vi "sync init.vi"(8 "error in (no error)":errorcluster, 9 "data allocations in":T1, 10 "shared memory configuration in":refnum<class "Shared Memory configuration.lvclass">, 11 "shared memory runtime in":refnum<class "Shared Memory runtime.lvclass">) -> (0 "error out":errorcluster, 1 "data allocations out":T1, 2 "shared memory configuration out":refnum<class "Shared Memory configuration.lvclass">, 3 "shared memory runtime out":refnum<class "Shared Memory runtime.lvclass">)   [LabVIEW 2014, in "Shared Memory runtime.lvclass"]
uses:
  Shared Memory runtime.lvclass
  configuration/Shared Memory configuration.lvclass
  <vilib>/NI/Tag Bus Module Framework/channel/data tables.ctl
  <vilib>/NI/Tag Bus/dictionary/data dictionary.lvclass
  <vilib>/NI/Tag Bus/dictionary table pair.ctl
  <vilib>/NI/Tag Bus/table/data table.ctl
  configuration/Shared Memory configuration.lvclass/Shared Memory configuration.ctl
  controls/sync data.ctl
  controls/semaphore data.ctl
  <vilib>/NI/NI Linux RT IPC/POSIX Threads/Classes/Semaphore/Controls/reference.ctl
  <vilib>/NI/NI Linux RT IPC/POSIX Threads/Classes/Semaphore/Semaphore.lvclass
  <vilib>/NI/NI Linux RT IPC/Shared Memory/Classes/Shared Memory/Public/Controls/reference.ctl
  <vilib>/NI/NI Linux RT IPC/Shared Memory/Classes/Shared Memory/Shared Memory.lvclass
  controls/sync timing indices.ctl
  controls/sync timing pointers.ctl
  Shared Memory runtime.lvclass/Shared Memory runtime.ctl
  configuration/Read sync enable.vi
  configuration/Read sync shm name.vi
  configuration/Read include start time.vi
  configuration/Read sync start of cycle.vi
  configuration/Read sync end of cycle.vi
  configuration/Read sync timeout seconds.vi
  Write sync data.vi
  <vilib>/NI/Tag Bus/table/data table.lvlib
  <vilib>/NI/Tag Bus/tag bus.lvlib
  <vilib>/NI/Tag Bus Module Framework/channel/TBM channel.lvclass
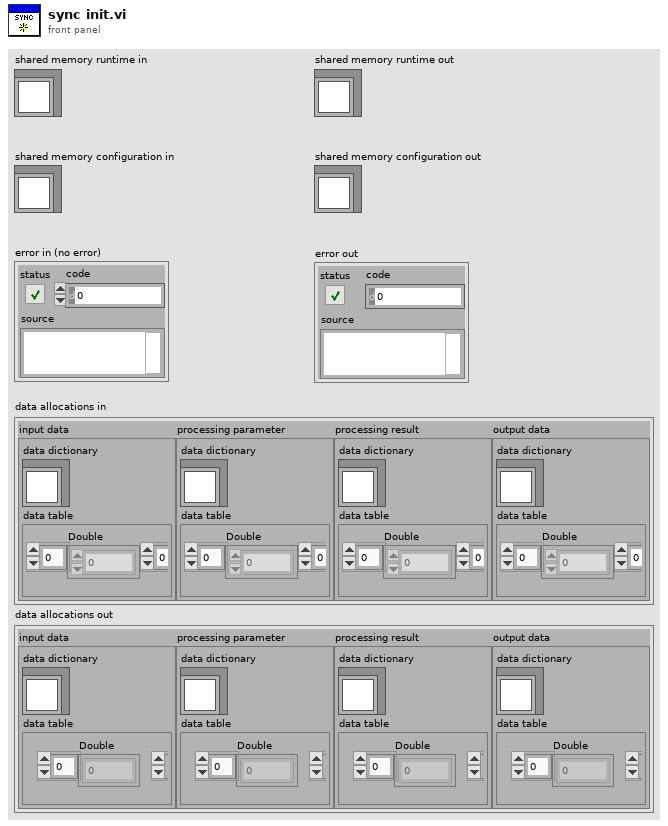
[diagram p1: front panel]
types:
  T1 = typedef "TBM channel.lvclass/data tables.ctl" = cluster{"input data":T2, "processing parameter":T2, "processing result":T2, "output data":T2}
  T2 = typedef "tag bus.lvlib/dictionary table pair.ctl" = cluster{"data dictionary":refnum<class "data dictionary.lvclass">, "data table":T3}
  T3 = typedef "tag bus.lvlib/data table.lvlib/data table.ctl" = cluster{"Double":dbl[], "Single":sgl[], "I64":i64[], "I32":i32[], "I16":i16[], "I8":i8[], "U64":u64[], "U32":u32[], "U16":u16[], "U8":u8[], "Boolean":bool[], "String":string[], "Array of Double":cluster{"DBL Array":dbl[]}[], "Array of Single":cluster{"SGL Array":sgl[]}[], "Array of I64":cluster{"I64 Array":i64[]}[], "Array of I32":cluster{"I32 Array":i32[]}[], "Array of I16":cluster{"I16 Array":i16[]}[], "Array of I8":cluster{"I8 Array":i8[]}[], "Array of U64":cluster{"U64 Array":u64[]}[], "Array of U32":cluster{"U32 Array":u32[]}[], "Array of U16":cluster{"U16 Array":u16[]}[], "Array of U8":cluster{"U8 Array":u8[]}[], "Array of Boolean":cluster{"Boolean Array":bool[]}[], "Array of String":cluster{"String Array":string[]}[]}
  T4 = typedef "Shared Memory configuration.lvclass/sync item.ctl" = cluster{"mechanism":T5, "name":string}
  T5 = typedef "Shared Memory configuration.lvclass/sync mechanism.ctl" = enum16{"Semaphore"}
  T6 = typedef "Shared Memory runtime.lvclass/sync data.ctl" = cluster{"semaphores soc":T7[], "semaphores eoc":T7[], "timeout":dbl, "enabled":bool, "sync shared memory":T9, "publish timing":bool, "timing indices":T10, "timing pointers":T11}
  T7 = typedef "Shared Memory runtime.lvclass/semaphore data.ctl" = cluster{"semaphore":T8, "name":string}
  T8 = typedef "POSIX Threads.lvlib/Semaphore.lvclass/reference.ctl" = refnum<data-value>
  T9 = typedef "Shared Memory.lvlib/Shared Memory.lvclass/reference.ctl" = refnum<data-value>
  T10 = typedef "Shared Memory runtime.lvclass/sync timing indices.ctl" = cluster{"start time index":i32}
  T11 = typedef "Shared Memory runtime.lvclass/sync timing pointers.ctl" = cluster{"start sec ptr":u64, "start nsec ptr":u64}
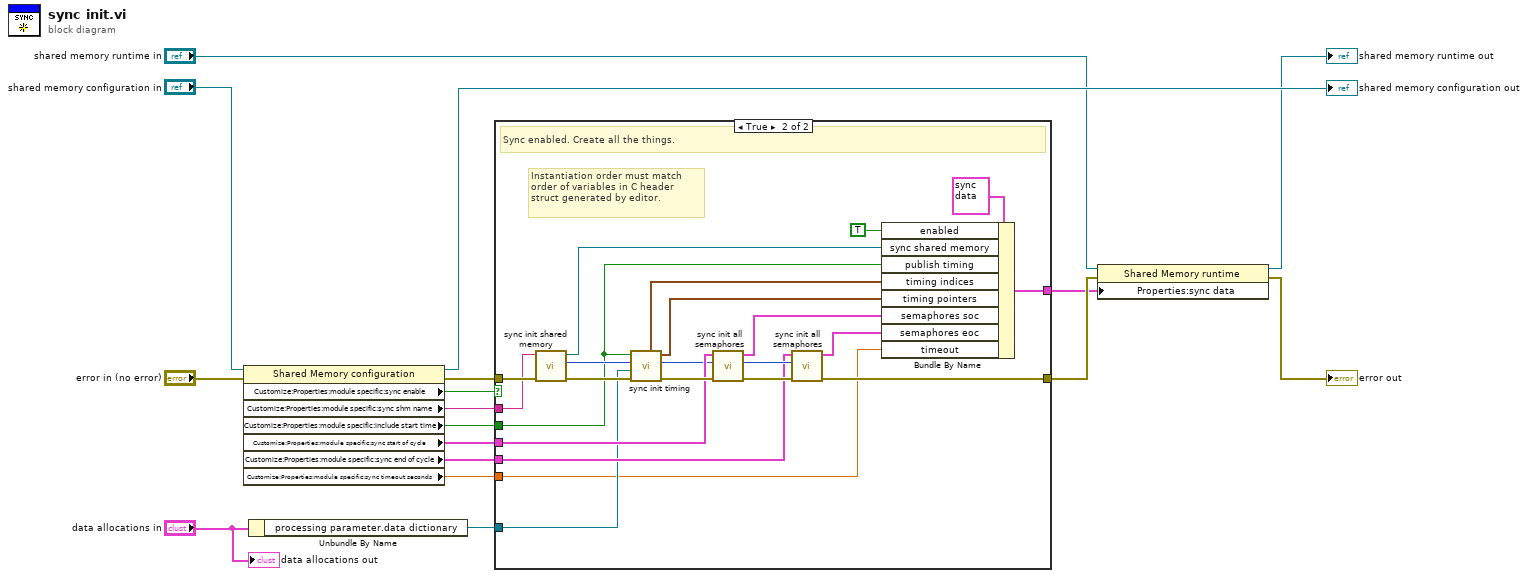
[diagram p0: block diagram]
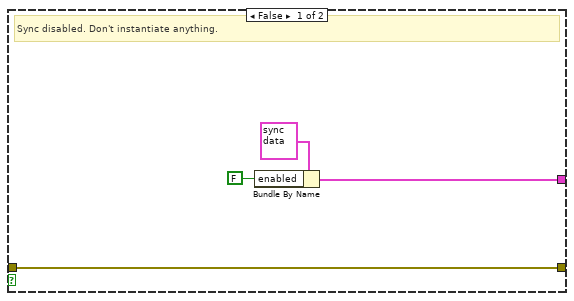
[diagram p2: hidden frame]
diagram:
  n1 = property class="Shared Memory configuration"(reference="shared memory configuration in", error in="error in (no error)") -> (reference out=→"shared memory configuration out":refnum<class "Shared Memory configuration.lvclass">, error out=w12:errorcluster, "Customize:Properties:module specific:sync enable"=w7:bool, "Customize:Properties:module specific:sync shm name"=w10:string, "Customize:Properties:module specific:include start time"=w3:bool, "Customize:Properties:module specific:sync start of cycle"=w9:T4[], "Customize:Properties:module specific:sync end of cycle"=w8:T4[], "Customize:Properties:module specific:sync timeout seconds"=w4:dbl)
  n2 = Unbundle By Name("data allocations in") -> ("processing parameter.data dictionary"=w1:refnum<class "data dictionary.lvclass">)
  n3 = case shown="True" w7 {
    tunnel: w12 -> [w21 w43]
    tunnel: [w21 w32] -> w17
    tunnel: w10 -> [_ w42]
    tunnel: w9 -> [_ w29]
    tunnel: w8 -> [_ w34]
    tunnel: [w18 w40] -> w6
    tunnel: w4 -> [_ w22]
    tunnel: w3 -> [_ w26]
    tunnel: w1 -> [_ w27]
    frame False {
      # "Sync disabled. Don't instantiate anything."
      n4 = Bundle By Name(cluster=T6 {"semaphores soc"=[], "semaphores eoc"=[], "timeout"=0.0, "enabled"=FALSE, "sync shared memory"=refnum, "publish timing"=FALSE, "timing indices"={"start time index"=0}, "timing pointers"={"start sec ptr"=0, "start nsec ptr"=0}} ("sync data"), "enabled"=FALSE) -> (w18:T6)
    }
    frame True {
      # "Instantiation order must match order of variables in C header struct generated by editor."
      # "Sync enabled. Create all the things."
      n5 = call "sync init shared memory.vi"("error in (no error)"=w43, "sync shm name"=w42) -> ("error out"=w28:errorcluster, "pointer to shared memory"=w31:u64, "shared memory out"=w38:T9)  [unwired: 7 in]
      n6 = call "sync init timing.vi"("error in (no error)"=w28, "data dictionary in"=w27, "pointer in"=w31, "publish timing?"=w26) -> ("error out"=w30:errorcluster, "pointer out"=w23:u64, "timing pointers"=w24:T11, "timing indices"=w25:T10)  [unwired: 4 in]
      n7 = call "sync init all semaphores.vi"("error in (no error)"=w30, "pointer to shared memory"=w23, "sync items"=w29) -> ("error out"=w36:errorcluster, "offset pointer out"=w35:u64, "initialized semaphores"=w37:T7[])  [unwired: 6 in]
      n8 = call "sync init all semaphores.vi"("error in (no error)"=w36, "pointer to shared memory"=w35, "sync items"=w34) -> ("error out"=w32:errorcluster, "initialized semaphores"=w33:T7[])  [unwired: 6 in, 1 out]
      n9 = Bundle By Name(cluster=T6 {"semaphores soc"=[], "semaphores eoc"=[], "timeout"=0.0, "enabled"=FALSE, "sync shared memory"=refnum, "publish timing"=FALSE, "timing indices"={"start time index"=0}, "timing pointers"={"start sec ptr"=0, "start nsec ptr"=0}} ("sync data"), "enabled"=TRUE, "sync shared memory"=w38, "publish timing"=w26, "timing indices"=w25, "timing pointers"=w24, "semaphores soc"=w37, "semaphores eoc"=w33, "timeout"=w22) -> (w40:T6)
    }
  }
  n10 = property class="Shared Memory runtime"(reference="shared memory runtime in", error in=w17, "Properties:sync data"=w6) -> (reference out=→"shared memory runtime out":refnum<class "Shared Memory runtime.lvclass">, error out=→"error out":errorcluster)
  "data allocations out" <- "data allocations in"
